vi "Tree selection apply selection.vi"(8 "error in (no error)":errorcluster, 10 "Selection States":bool[](array[boolean]), 11 "Loop data":T1) -> (0 "error out":errorcluster, 3 "Loop data":T1)   [LabVIEW 2020, in "UI_ItemSelect.lvlib"]
uses:
  UI_ItemSelect.lvlib
  Tree item select loop data.ctl
  Item select ref type.ctl
  Tree item loop data.ctl
  Tree item selection indices.ctl
  checkbox state.ctl
  item select tree lock states.ctl
  <userlib>/Blue Origin/DeferPanelUpdates_OpenSource/SubVIs/defer panel updates Controlref step1.vi
  <userlib>/Blue Origin/DeferPanelUpdates_OpenSource/SubVIs/defer panel updates step2.vi
  <userlib>/Blue Origin/DeferPanelUpdates_OpenSource/Defer Panel Updates OpenSource.lvlib
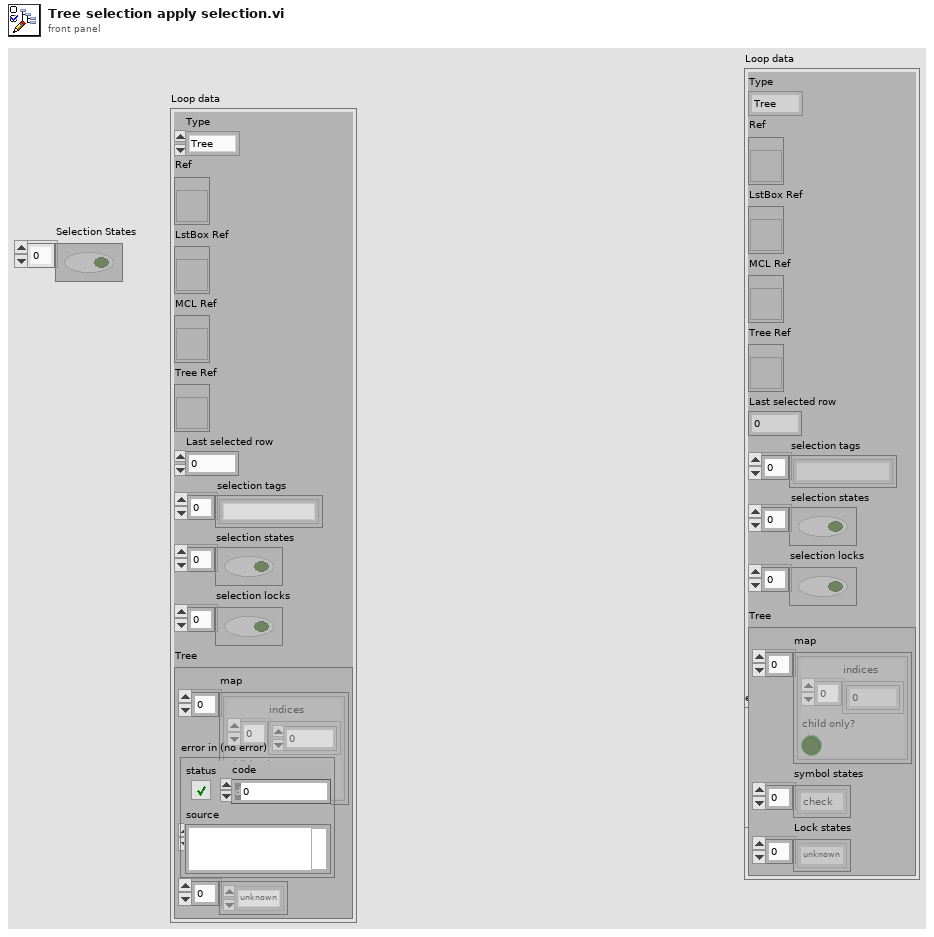
[diagram p1: front panel]
types:
  T1 = typedef "UI_ItemSelect.lvlib/Tree item select loop data.ctl" = cluster{"Type":T2, "Ref":refnum<vi>, "LstBox Ref":refnum<vi>, "MCL Ref":refnum<vi>, "Tree Ref":refnum<vi>, "Last selected row":i32, "selection tags":string[], "selection states":bool[], "selection locks":bool[], "Tree":T3}
  T2 = typedef "UI_ItemSelect.lvlib/Item select ref type.ctl" = enum16{"Tree", "MCL", "ListBox"}
  T3 = typedef "UI_ItemSelect.lvlib/Tree item loop data.ctl" = cluster{"map":T4[], "symbol states":T5[], "Lock states":T6[]}
  T4 = typedef "UI_ItemSelect.lvlib/Tree item selection indices.ctl" = cluster{"indices":i32[], "child only?":bool}
  T5 = typedef "UI_ItemSelect.lvlib/checkbox state.ctl" = enum16{"unknown", "check", "some", "no check"}
  T6 = typedef "UI_ItemSelect.lvlib/item select tree lock states.ctl" = enum16{"unknown", "locked", "unlocked"}
  T7 = typedef "Defer Panel Updates OpenSource.lvlib/defer panel updates data.ctl" = cluster{"Owning VI":refnum<vi>, "Front Panel":refnum<vi>, "performed?":bool}
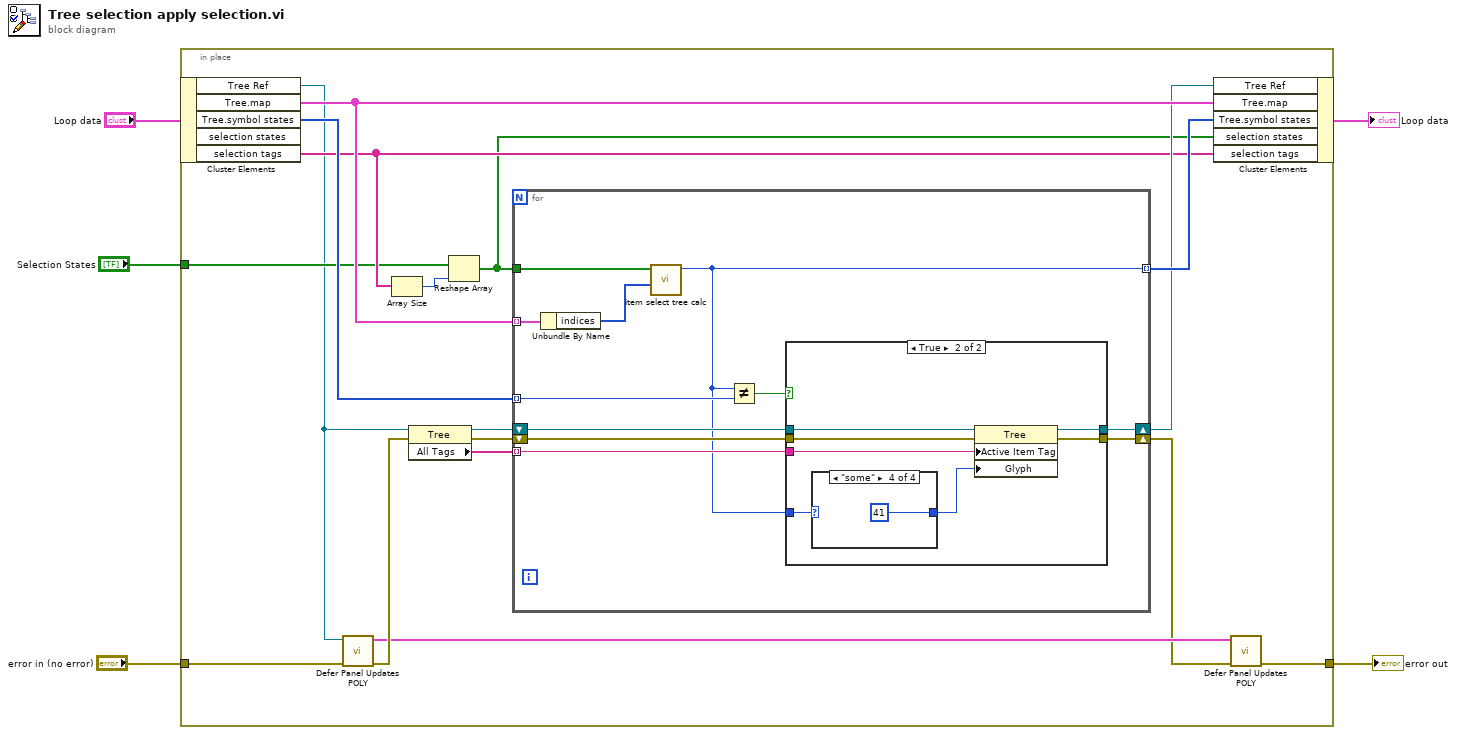
[diagram p0: block diagram]
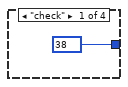
[diagram p3: hidden frame]
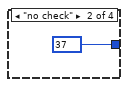
[diagram p4: hidden frame]
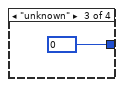
[diagram p5: hidden frame]
diagram:
  n1 = in-place {
    in-place-border: "error in (no error)" -> [w10]
    in-place-border: [w6] -> w2
    in-place-border: "Selection States" -> [w13]
    n2 = in-place-cluster #1("Loop data") -> ("Tree Ref"=w11:refnum<vi>, "Tree.map"=w21:T4[], "Tree.symbol states"=w20:T5[], "selection tags"=w15:string[])  [unwired: 1 out]
    n3 = call-poly <userlib>:"Defer Panel Updates POLY.vi"("error in (no error)"=w10, "control reference"=w11) -> ("error out"=w9:errorcluster, "Refs"=w8:T7)  [unwired: 8 in]
    n4 = Array Size(array=w15) -> (size(s)=w14:i32)
    n5 = property class="Tree"(reference=w11, error in=w9) -> (reference out=w19:refnum<vi>, error out=w17:errorcluster, "All Tags"=w18:string[])
    n6 = Reshape Array(w13, w14) -> (w12:bool[])
    n7 = for {
      tunnel: w21 -> [w33] mode=indexing
      tunnel: w12 -> [w23]
      tunnel: [w25] -> w22 mode=indexing
      tunnel: w20 -> [w30] mode=indexing
      tunnel: w18 -> [w31] mode=indexing
      shift-right: [w27] -> w7
      shift-left: w17 -> [w28]
      shift-right: [w26] -> w16
      shift-left: w19 -> [w32]
      n8 = Unbundle By Name(w33) -> ("indices"=w24:i32[])
      n9 = call "item select tree calc.vi"("indices"=w24, "selection states"=w23) -> ("symbol state"=w25:T5)  [unwired: 9 in]
      n10 = Not Equal?(x=w25, y=w30) -> (x != y?=w29:bool)
      n11 = case shown="True" w29 {
        tunnel: w32 -> [w34 w42]
        tunnel: w31 -> [_ w41]
        tunnel: w25 -> [_ w40]
        tunnel: w28 -> [w35 w38]
        tunnel: [w35 w37] -> w27
        tunnel: [w34 w36] -> w26
        frame False {
        }
        frame True {
          n12 = case shown="\"some\"" w40 {
            tunnel: [38 37 0 41] -> w39
            frame "check" {
            }
            frame "no check" {
            }
            frame "unknown" {
            }
            frame "some" {
            }
          }
          n13 = property class="Tree"(reference=w42, error in=w38, "Active Item Tag"=w41, "Glyph"=w39) -> (reference out=w36:refnum<vi>, error out=w37:errorcluster)
        }
      }
    }
    n14 = in-place-cluster #1("Tree Ref"=w16, "Tree.map"=w21, "Tree.symbol states"=w22, "selection states"=w12, "selection tags"=w15) -> (→"Loop data":T1)
    n15 = call-poly <userlib>:"Defer Panel Updates POLY.vi"("error in (no error)"=w7, "Refs"=w8) -> ("error out"=w6:errorcluster)  [unwired: 9 in]
  }
  "error out" <- w2
